vi "Voltage_current_test.vi"() -> ()   [LabVIEW 2017]
uses:
  <vilib>/Utility/error.llb/DialogType.ctl
  <vilib>/DAQmx/read.llb/DAQmx Read (Analog 2D DBL NChan NSamp).vi
  <vilib>/DAQmx/read.llb/DAQmx Read (Analog 1D Wfm NChan NSamp).vi
  <vilib>/DAQmx/write.llb/DAQmx Write (Analog DBL 1Chan 1Samp).vi
  <vilib>/DAQmx/create/channels.llb/DAQmx Create Channel (AO-Voltage-Basic).vi
  <vilib>/DAQmx/create/channels.llb/DAQmx Create Channel (AI-Voltage-Basic).vi
  <vilib>/DAQmx/configure/timing.llb/DAQmx Timing (Sample Clock).vi
  <vilib>/DAQmx/configure/trigger.llb/DAQmx Start Trigger (None).vi
  <vilib>/DAQmx/miscellaneous.llb/DAQmx Fill In Error Info.vi
  <resource>/objmgr/daqmx.rc
panel:
  in  "Stop Voltage Output, V":dbl=0.5
  in  "Number of points":i32=200
  in  "Rsh":dbl=98.2 format="%0.1f"
  out "Average":dbl=-3.982433458528967e-05
  in  "samples per channel":i32=200000
  in  "rate":dbl=100000.0 format="%0.0f"
  out "MSE":dbl=0.0019468985949147193
  out "size of buffer":i32=9984
  out "size(s)":i32=200
  out "Ush.Min":dbl=-0.5
  out "Ush.Max":dbl=0.5
  out "U.Min":dbl=-0.2
  out "U.Max":dbl=0.2
  in  "Start Voltage Output, V":dbl=-0.5
  in  "ms to wait":u32=100
  out "AO.Max":dbl=0.5
  out "AO.Min":dbl=-0.5
  in  "Error (in)":errorcluster
  in  "stop":bool
  out "SpectrumGraph":cluster{dbl[], dbl[]}(graph)={[-0.11227699865080601, -0.11219631251702926, -0.1110375342644668, -0.1098959907862774, -0.10879200578105087, -0.10765484359322787, -0.10655129683069368, -0.1054163644166972, -0.10426965442042564, -0.10316647412156116, -0.10201968439244481, -0.10091651958050508, -0.0997796308447607, -0.09864611100924825, -0.09754331382966656, -0.09639339626879585, -0.09527088002298219, -0.09409529518804473, -0.0928779508122345, -0.09166194369892135, -0.08917955963403298, -0.08654392981010957, -0.08560066899536561, -0.08452667685927212, -0.08345132483671222, -0.08236129806228541, -0.08128284936856425, -0.08018384789520756, -0.07908900657048462, -0.07802040770362137, -0.0769258827852659, -0.07584595761874936, -0.0747473511983118, -0.07365172154559965, -0.07257081627083269, -0.07147695977476184, -0.07040700941389362, -0.06930931538673835, -0.06820832518604475, -0.06712332670028925, -0.06602226651202146, -0.06495116311008292, -0.06384301749522095, -0.0627421378485943, -0.06166785284646776, -0.06056546518761769, -0.05949238648730333, -0.05837886878134868, -0.05730438495812015, -0.05619667069823077, -0.0550968521882794, -0.054017221908244886, -0.052921479767432285, -0.05184898524460873, -0.050740334980480375, -0.049639379535985656, -0.048555864026473015, -0.04745303606936762, -0.046365635930505314, -0.04527488873324592, -0.044176621951271165, -0.0431034977668357, -0.04199385234144701, -0.040920708921241326, -0.039813667134871195, -0.03871268124882551, -0.03762323649494599, -0.03653292218912251, -0.03546274607231973, -0.03435872014950309, -0.03324899590046898, -0.0321693833397791, -0.03106720632098697, -0.02998875433713212, -0.028885590157831605, -0.02778322644601457, -0.026707066388704633, -0.02560560812138877, -0.02451852206319557, -0.02341289462175359, -0.022312059740193818, -0.021235011051728644, -0.02013331197424583, -0.01905866463950425, -0.017954258969894558, -0.016837881666835888, -0.015763552090108667, -0.014664099149127264, -0.013590861428849505, -0.01248268980413928, -0.011380651945878135, -0.010304459022325116, -0.009190784043806847, -0.008118338935183461, -0.0070098439477931955, -0.0059086605317368495, -0.004834792218353594, -0.0037314289208216765, -0.0026577369969337026, -0.0015499792081472283, -0.0004503701378675076, 0.0006309937803072015, 0.0017386367363273509, 0.002813200126482827, 0.003914267940233872, 0.004991987496824608, 0.00609534019654466, 0.0071983561512158675, 0.008271425123778675, 0.009383268338301363, 0.010455997744464972, 0.011567565797297646, 0.012669105413192992, 0.01374596956328598, 0.014846941968856685, 0.015920901953368063, 0.01702773588065364, 0.018141542160538537, 0.019213581347042458, 0.020315375160029518, 0.021394247033860832, 0.02250134986741634, 0.02360331585452807, 0.0246896357335775, 0.025779500992563268, 0.026865203559265624, 0.02797061971138625, 0.029071220275376584, 0.03015403905272116, 0.031255926451088545, 0.032330516151466565, 0.033433380000035, 0.034534516828177465, 0.035623413820463044, 0.0367264010177051, 0.03779806824906324, 0.03892390155083866, 0.04001470502018629, 0.041089829666504187, 0.04218979072822027, 0.04326576923509265, 0.04438328579995733, 0.04549038106457023, 0.04656788469303866, 0.04766711521151217, 0.048739326863020606, 0.0498446266466979, 0.05094582383754943, 0.05202717532540858, 0.05314391769579876, 0.05421737876080723, 0.05532938657658881, 0.0564284800450863, 0.05750254973103692, 0.05860717382111526, 0.05967933168876977, 0.06079484570445765, 0.06190063766864651, 0.0629704622366188, 0.06407384680568495, 0.06515403444475577, 0.0662535941506172, 0.06732955186543266, 0.06843700761815802, 0.06953987525063422, 0.0706276727337431, 0.07173201681061904, 0.07280466276759895, 0.07391202986982796, 0.07501767710575971, 0.07609180407108769, 0.077192538811952, 0.07828175267646821, 0.07938884870891301, 0.08049362943808833, 0.08156782621539194, 0.08267359324682853, 0.08374478305045753, 0.08484827725095598, 0.0859531162650569, 0.0870415082701936, 0.0881433456530262, 0.08921769253931768, 0.0903269120261113, 0.09143042355096091, 0.09250694767641957, 0.09360855346389012, 0.09468145243672565, 0.09579494714192201, 0.09690322891092021, 0.09798088942176283, 0.09908419059906141, 0.10015929625879326, 0.10126372419769593, 0.10236358981277881, 0.10344237387968673, 0.10455359332971775, 0.10563377646273668, 0.10673843740341372, 0.10784957310764727], [-0.0034359701165033764, -0.0034334812365722, -0.003397937289119619, -0.003363021877223209, -0.003329280865867832, -0.003294503654458856, -0.003260701675515121, -0.003225931334395744, -0.003190868501585349, -0.003157154302953141, -0.0031220504276250126, -0.0030882601710504683, -0.0030534978230179546, -0.003018791659377652, -0.002985021518667652, -0.00294985583933235, -0.00291547312677725, -0.002879492313869344, -0.0028422398210563252, -0.0028049743033878665, -0.0027290488104605034, -0.0026480037320946673, -0.0026191009094931905, -0.0025861737347635597, -0.0025532744613464453, -0.002519947764299584, -0.0024870294605233425, -0.002453364985081822, -0.0024198489796247616, -0.002387203024130146, -0.0023536972938074433, -0.0023206831454535165, -0.0022870708492618284, -0.0022535553114736567, -0.0022205080028002426, -0.0021869435171406773, -0.002154267394470466, -0.002120676790503153, -0.002086984606982967, -0.002053788828862956, -0.0020200679141789126, -0.001987263988097909, -0.0019533222161346128, -0.0019196472216249962, -0.001886804247881894, -0.0018530893982665391, -0.0018202907709804355, -0.001786159959954426, -0.0017532920362669185, -0.0017194658771953275, -0.0016857338767370027, -0.001652689472666745, -0.0016191588108596339, -0.001586355834973737, -0.001552457574781964, -0.0015187033871081408, -0.0014855963416983173, -0.0014519014792530194, -0.0014185735120573202, -0.0013852266200080267, -0.0013515909121641022, -0.0013187598277836698, -0.0012847824858589101, -0.001251937205359635, -0.001218050661269074, -0.001184378944414725, -0.001151081430863748, -0.0011176951997681583, -0.001084940829454201, -0.0010511256730461305, -0.0010172113140042333, -0.0009841388072280614, -0.0009504381432089305, -0.0009174387737222211, -0.0008836789330344166, -0.0008499270790267385, -0.0008170840146479927, -0.0007833390822159676, -0.0007501227581971934, -0.0007162731962949148, -0.0006825960536106279, -0.0006496806298016717, -0.0006158915578716437, -0.0005829995997222753, -0.0005492286312683955, -0.0005150661925209235, -0.0004822080403691795, -0.00044849944851975784, -0.0004156298896395494, -0.0003817215580463585, -0.0003480125883069288, -0.0003151743150818938, -0.0002810451112935865, -0.0002482756199767183, -0.00021429598892350342, -0.00018062315645895228, -0.00014777922261907466, -0.00011397432189183147, -8.109219601232683e-05, -4.723657521894207e-05, -1.359877912662274e-05, 1.94989733097235e-05, 5.339320397002653e-05, 8.627902587406503e-05, 0.00012001299991695115, 0.0001529433118020672, 0.00018671105205403848, 0.00022042460006405413, 0.0002533007233442487, 0.00028734093085948587, 0.0003201458450368361, 0.00035407868700219235, 0.0003878782514198857, 0.00042082159960751624, 0.0004545228323934206, 0.00048740507161829734, 0.0005211534201252651, 0.0005552951262743767, 0.0005880895068965784, 0.0006218595254034199, 0.000654887061862146, 0.0006887779372489097, 0.0007224538264404176, 0.0007557163501634893, 0.000789067402547219, 0.0008223257485797882, 0.0008560340312464532, 0.0008897637060036905, 0.0009228449229764379, 0.0009565743758726721, 0.000989410799933107, 0.0010232423691113129, 0.0010569745726820457, 0.0010902531917189998, 0.0011240163594060536, 0.0011568329466930566, 0.0011912200140887005, 0.0012246362043661304, 0.0012574902719893134, 0.0012911640824512564, 0.0013240713062982522, 0.0013582968659198685, 0.0013921215764981247, 0.001425141062923694, 0.001458727031649257, 0.001491609293721653, 0.001525403417514198, 0.0015591025222435522, 0.0015921449375247317, 0.0016263269732749992, 0.0016592057435537639, 0.0016932131099534598, 0.001726830989001125, 0.0017597067111599128, 0.0017934893708655526, 0.001826341810573146, 0.0018604723679566222, 0.001894241396717838, 0.0019270456460640513, 0.001960821352723349, 0.0019937631756405073, 0.0020274979506900268, 0.0020604075490265276, 0.002094264484801711, 0.002128038209177847, 0.0021613328927250096, 0.0021950765786994896, 0.0022279284428932014, 0.002261828197059583, 0.0022956503482628545, 0.002328532603270199, 0.00236219118564215, 0.002395524431933338, 0.002429351348980483, 0.0024631731623826303, 0.0024960279897970725, 0.0025298611339761223, 0.0025626174430144776, 0.0025963710909140372, 0.002630231218322425, 0.0026635006685309247, 0.0026972077272103398, 0.00273008696315015, 0.002764010814667285, 0.002797747887573997, 0.0028307375890992185, 0.0028644020376768554, 0.002897235108452893, 0.002931378080248272, 0.0029651883836858376, 0.002998208925923221, 0.003031969398106626, 0.0030647813290643547, 0.0030986157750069318, 0.003132283530124602, 0.0031652737347853924, 0.003199264945236897, 0.0032323321050158325, 0.0032660899247958443, 0.0033000991183870666]}
  out "error out":errorcluster
  in  "DAQ channel In Voltage Output":tag="DAQ6363/ao0"
  in  "DAQ channel In Voltage U":tag="DAQ6363/ai5"
  in  "DAQ channel In Voltage Ush":tag="DAQ6363/ai4"
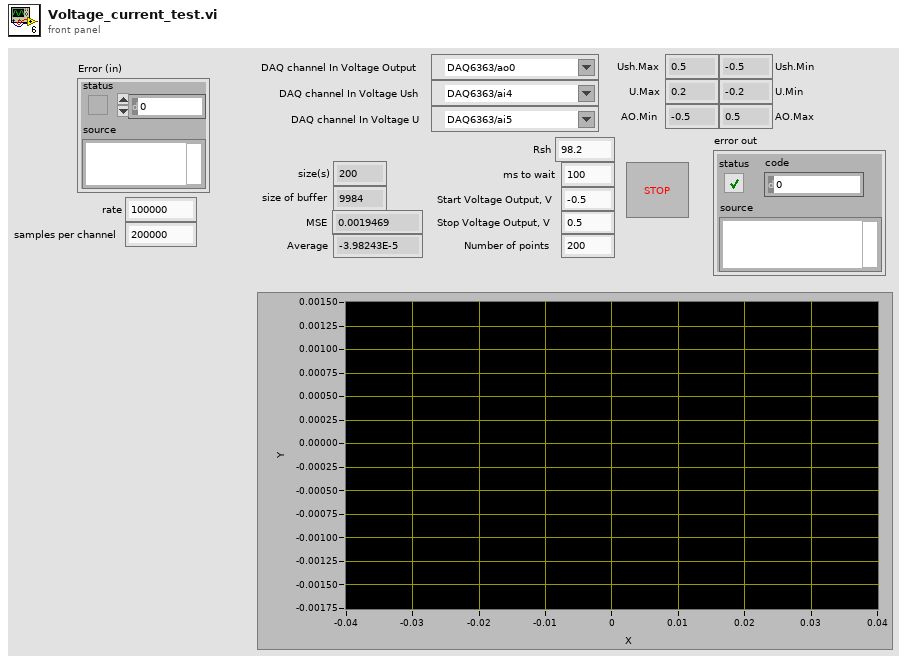
[diagram p1: front panel]
types:
  T1 = typedef "DialogType.ctl" = u16
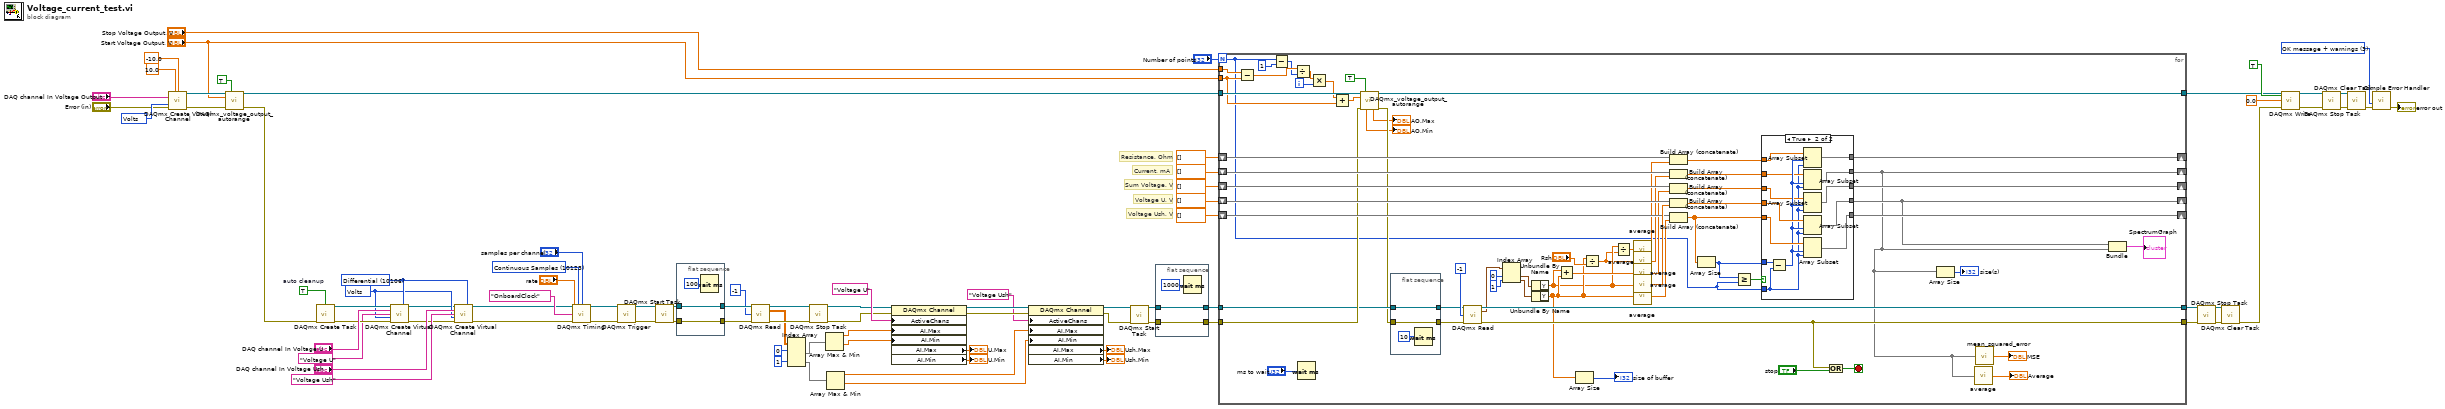
[diagram p0: block diagram]
diagram:
  w56 = 10348 items=["Volts"=10348, "From Custom Scale"=10065] ("units")
  w77 = TRUE  # auto cleanup
  w81 = T1 3 items=["no dialog", "OK message", "continue or stop message", "OK message + warnings", "continue/stop + warnings"] ("type of dialog (OK msg:1)")
  w85 = 10123 items=["Finite Samples"=10178, "Continuous Samples"=10123, "Hardware Timed Single Point"=12522] ("sample mode")
  w19 = 10106 items=["Default"=-1, "RSE"=10083, "NRSE"=10078, "Differential"=10106, "Pseudodifferential"=12529] ("input terminal configuration")
  w18 = 10348 items=["Volts"=10348, "From Custom Scale"=10065] ("units")
  # "Sum Voltage, V"
  # "Current, mA"
  # "Resistance, Ohm"
  # "Voltage Ush, V"
  # "Voltage U, V"
  n1 = call-poly <vilib>:"DAQmx Create Virtual Channel.vi"("maximum value"=10.0, "minimum value"=-10.0, "physical channels"="DAQ channel In Voltage Output", "units"=w56, "error in"="Error (in)") -> ("task out"=w5:refnum<k21>, "error out"=w6:errorcluster)  [unwired: 9 in]
  n2 = call "DAQmx_voltage_output_autorange.vi"("DAQ task Voltage Output in"=w5, "Bipolar"=TRUE, "Voltage Output, V"="Start Voltage Output, V", "error in (no error)"=w6) -> ("DAQ task Voltage Output out"=w4:refnum<k21>, "error out"=w3:errorcluster)  [unwired: 8 in, 2 out]
  n3 = call <vilib>:"DAQmx Create Task.vi"("auto cleanup"=w77, "error in"=w3) -> ("task out"=w76:refnum<k21>, "error out"=w75:errorcluster)  [unwired: 12 in]
  n4 = call-poly <vilib>:"DAQmx Create Virtual Channel.vi"("task in"=w76, "input terminal configuration"=w19, "physical channels"="DAQ channel In Voltage U", "name to assign"="Voltage U", "units"=w18, "error in"=w75) -> ("task out"=w13:refnum<k21>, "error out"=w12:errorcluster)  [unwired: 8 in]
  n5 = call-poly <vilib>:"DAQmx Create Virtual Channel.vi"("task in"=w13, "input terminal configuration"=w19, "physical channels"="DAQ channel In Voltage Ush", "name to assign"="Voltage Ush", "units"=w18, "error in"=w12) -> ("task out"=w73:refnum<k21>, "error out"=w72:errorcluster)  [unwired: 8 in]
  n6 = call-poly <vilib>:"DAQmx Timing.vi"("task/channels in"=w73, "sample mode"=w85, "samples per channel"="samples per channel", "rate"="rate", "source"=tag "OnboardClock", "error in"=w72) -> ("task out"=w71:refnum<k21>, "error out"=w70:errorcluster)  [unwired: 8 in]
  n7 = call-poly <vilib>:"DAQmx Trigger.vi"("task/channels in"=w71, "error in"=w70) -> ("task out"=w31:refnum<k21>, "error out"=w30:errorcluster)  [unwired: 12 in]
  n8 = call <vilib>:"DAQmx Start Task.vi"("task/channels in"=w31, "error in"=w30) -> ("task out"=w40:refnum<k21>, "error out"=w38:errorcluster)  [unwired: 12 in]
  n9 = flat-sequence {
    tunnel: w38 -> [w89]
    tunnel: [w89] -> w39
    tunnel: w40 -> [w88]
    tunnel: [w88] -> w41
    frame #0 {
      n10 = Wait (ms)(milliseconds to wait=u32 100) -> ()  [unwired: 1 out]
    }
  }
  n11 = call-poly <vilib>:"DAQmx Read.vi"("task/channels in"=w41, "number of samples per channel"=-1, "error in"=w39) -> ("task out"=w35:refnum<k21>, "data"=w34:dbl[][], "error out"=w36:errorcluster)  [unwired: 10 in]
  n12 = Index Array(array=w34, index (row) #1=0 ("index"), index (row) #2=1 ("index")) -> (element #1=w42:dbl[], element #2=w43:dbl[])  [unwired: 2 in]
  n13 = call <vilib>:"DAQmx Stop Task.vi"("task/channels in"=w35, "error in"=w36) -> ("task out"=w29:refnum<k21>, "error out"=w28:errorcluster)  [unwired: 12 in]
  n14 = Array Max & Min(array=w42) -> (max value=w27:dbl, min value=w26:dbl)  [unwired: 2 out]
  n15 = Array Max & Min(array=w43) -> (max value=w17:dbl, min value=w16:dbl)  [unwired: 2 out]
  n16 = property class="DAQmx Channel"(reference=w29, error in=w28, "ActiveChans"="Voltage U", "AI.Max"=w27, "AI.Min"=w26) -> (reference out=w61:refnum<k21>, error out=w60:errorcluster, "AI.Max"=→"U.Max":dbl, "AI.Min"=→"U.Min":dbl)
  n17 = property class="DAQmx Channel"(reference=w61, error in=w60, "ActiveChans"="Voltage Ush", "AI.Max"=w17, "AI.Min"=w16) -> (reference out=w15:refnum<k21>, error out=w14:errorcluster, "AI.Max"=→"Ush.Max":dbl, "AI.Min"=→"Ush.Min":dbl)
  n18 = call <vilib>:"DAQmx Start Task.vi"("task/channels in"=w15, "error in"=w14) -> ("task out"=w23:refnum<k21>, "error out"=w22:errorcluster)  [unwired: 12 in]
  n19 = flat-sequence {
    tunnel: w22 -> [w92]
    tunnel: [w92] -> w24
    tunnel: w23 -> [w91]
    tunnel: [w91] -> w25
    frame #0 {
      n20 = Wait (ms)(milliseconds to wait=u32 1000) -> ()  [unwired: 1 out]
    }
  }
  n21 = for {
    N: "Number of points" -> [w98]
    tunnel: w25 -> [w112]
    tunnel: w24 -> [w113]
    tunnel: [w149] -> w69
    tunnel: [w155] -> w68
    tunnel: w4 -> [w116]
    tunnel: [w108] -> w54
    shift-right: [w118] -> _
    shift-left: dbl[] [] -> [w146]
    shift-right: [w119] -> _
    shift-left: dbl[] [] -> [w145]
    shift-right: [w94] -> _
    shift-left: dbl[] [] -> [w130]
    shift-right: [w93] -> _
    shift-left: dbl[] [] -> [w131]
    shift-right: [w120] -> _
    shift-left: dbl[] [] -> [w132]
    tunnel: "Stop Voltage Output, V" -> [w105]
    tunnel: "Start Voltage Output, V" -> [w100]
    i -> [w114]
    stop <- w96 stop-if-true
    n22 = Subtract(x=w105, y=w100) -> (x-y=w104:dbl)
    n23 = Subtract(x=w98, y=1) -> (x-y=w102:i32)
    n24 = Divide(x=w104, y=w102) -> (x/y=w115:dbl)
    n25 = Wait (ms)(milliseconds to wait="ms to wait") -> ()  [unwired: 1 out]
    n26 = Multiply(x=w115, y=w114) -> (x*y=w101:dbl)
    n27 = Add(x=w101, y=w100) -> (x+y=w99:dbl)
    n28 = call "DAQmx_voltage_output_autorange.vi"("DAQ task Voltage Output in"=w116, "Bipolar"=TRUE, "Voltage Output, V"=w99, "error in (no error)"=w113) -> ("DAQ task Voltage Output out"=w108:refnum<k21>, "AO.Min"=→"AO.Min":dbl, "AO.Max"=→"AO.Max":dbl, "error out"=w109:errorcluster)  [unwired: 8 in]
    n29 = flat-sequence {
      tunnel: w112 -> [w159]
      tunnel: [w159] -> w111
      tunnel: [w158] -> w110
      tunnel: w109 -> [w158]
      frame #0 {
        n30 = Wait (ms)(milliseconds to wait=u32 10) -> ()  [unwired: 1 out]
      }
    }
    n31 = call-poly <vilib>:"DAQmx Read.vi"("task/channels in"=w111, "number of samples per channel"=-1, "error in"=w110) -> ("task out"=w155:refnum<k21>, "data"=w154:waveform(dbl)[], "error out"=w149:errorcluster)  [unwired: 10 in]
    n32 = Index Array(array=w154, index #1=0 ("index"), index #2=1 ("index")) -> (element #1=w151:waveform(dbl), element #2=w150:waveform(dbl))
    n33 = Unbundle By Name(w151) -> ("Y"=w135:dbl[])
    n34 = Unbundle By Name(w150) -> ("Y"=w136:dbl[])
    n35 = Add(x=w135, y=w136) -> (x+y=w138:dbl[])
    n36 = Array Size(array=w136) -> (size(s)=→"size of buffer":i32)
    n37 = Divide(x=w136, y="Rsh") -> (x/y=w134:dbl[])
    n38 = Divide(x=w135, y=w134) -> (x/y=w133:dbl[])
    n39 = call "average.vi"("Array"=w133) -> ("Average"=w127:dbl)
    n40 = call "average.vi"("Array"=w134) -> ("Average"=w128:dbl)
    n41 = call "average.vi"("Array"=w138) -> ("Average"=w129:dbl)
    n42 = call "average.vi"("Array"=w135) -> ("Average"=w147:dbl)
    n43 = call "average.vi"("Array"=w136) -> ("Average"=w144:dbl)
    n44 = Build Array (concatenate)(w130, w127) -> (w124:dbl[])
    n45 = Build Array (concatenate)(w131, w128) -> (w125:dbl[])
    n46 = Build Array (concatenate)(w132, w129) -> (w126:dbl[])
    n47 = Build Array (concatenate)(w146, w147) -> (w143:dbl[])
    n48 = Build Array (concatenate)(w145, w144) -> (w123:dbl[])
    n49 = Array Size(array=w123) -> (size(s)=w141:i32)
    n50 = Greater Or Equal?(x=w141, y=w98) -> (x >= y?=w142:bool)
    n51 = case shown="True" w142 {
      tunnel: [w164 w177] -> w118
      tunnel: w143 -> [w164 w176]
      tunnel: w123 -> [w163 w174]
      tunnel: w141 -> [_ w175]
      tunnel: w98 -> [_ w168]
      tunnel: [w163 w173] -> w119
      tunnel: w126 -> [w160 w169]
      tunnel: w125 -> [w161 w170]
      tunnel: w124 -> [w162 w171]
      tunnel: [w160 w167] -> w120
      tunnel: [w161 w166] -> w93
      tunnel: [w162 w165] -> w94
      frame False {
      }
      frame True {
        n52 = Subtract(x=w175, y=w168) -> (x-y=w172:i32)
        n53 = Array Subset(array=w171, index=w172, length=w168) -> (w165:dbl[])
        n54 = Array Subset(array=w170, index=w172, length=w168) -> (w166:dbl[])
        n55 = Array Subset(array=w169, index=w172, length=w168) -> (w167:dbl[])
        n56 = Array Subset(array=w176, index=w172, length=w168) -> (w177:dbl[])
        n57 = Array Subset(array=w174, index=w172, length=w168) -> (w173:dbl[])
      }
    }
    n58 = Or(x=w149, y="stop") -> (x .or. y?=w96:bool)
    n59 = Array Size(array=w93) -> (size(s)=→"size(s)":i32)
    n60 = call "average.vi"("Array"=w93) -> ("Average"=→"Average":dbl)
    n61 = call "mean_squared_error.vi"("Array"=w93) -> ("Mean Squared Error"=→"MSE":dbl)
    n62 = Bundle(w118, w93) -> (→"SpectrumGraph":cluster{dbl[], dbl[]})  [unwired: 1 in]
  }
  n63 = call <vilib>:"DAQmx Stop Task.vi"("task/channels in"=w68, "error in"=w69) -> ("task out"=w83:refnum<k21>, "error out"=w84:errorcluster)  [unwired: 12 in]
  n64 = call <vilib>:"DAQmx Clear Task.vi"("task in"=w83, "error in"=w84) -> ("error out"=w53:errorcluster)  [unwired: 13 in]
  n65 = call-poly <vilib>:"DAQmx Write.vi"("task/channels in"=w54, "auto start"=TRUE, "data"=0.0, "error in"=w53) -> ("task out"=w66:refnum<k21>, "error out"=w67:errorcluster)  [unwired: 9 in, 1 out]
  n66 = call <vilib>:"DAQmx Stop Task.vi"("task/channels in"=w66, "error in"=w67) -> ("task out"=w79:refnum<k21>, "error out"=w80:errorcluster)  [unwired: 12 in]
  n67 = call <vilib>:"DAQmx Clear Task.vi"("task in"=w79, "error in"=w80) -> ("error out"=w52:errorcluster)  [unwired: 13 in]
  n68 = call <vilib>:"Simple Error Handler.vi"("type of dialog (OK msg:1)"=w81, "error in (no error)"=w52) -> ("error out"=→"error out":errorcluster)  [unwired: 3 in, 4 out]
